vi "Write experiments.vi"(2 "error in (no error)":errorcluster, 3 "Experiments":refnum<class "Experiment.lvclass">[](array[class]), 4 "Experiments_group.lvclass in":refnum<class "Experiments_group.lvclass">) -> (0 "error out":errorcluster, 1 "Experiments_group.lvclass out":refnum<class "Experiments_group.lvclass">)   [LabVIEW 2019, in "Experiments_group.lvclass"]
uses:
  Experiments_group.lvclass
  Experiment.lvclass
  Experiments_group.lvclass/Experiments_group.ctl
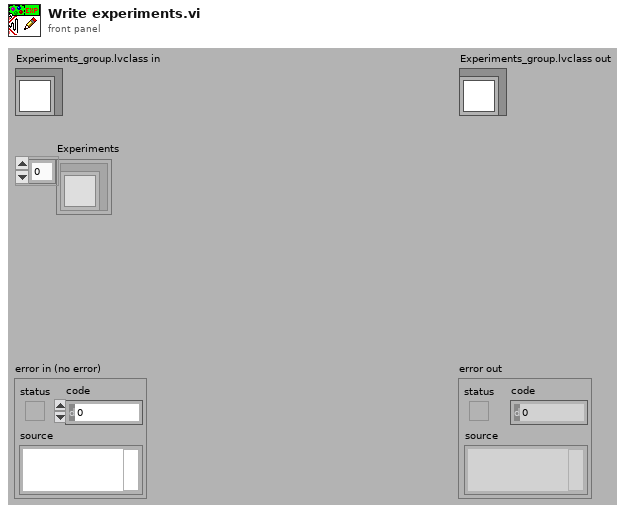
[diagram p1: front panel]
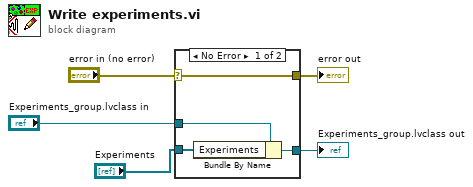
[diagram p0: block diagram]
diagram:
  n1 = case shown="No Error" "error in (no error)" {
    selector: "error in (no error)" -> [w9 w10]
    tunnel: [w9 w10] -> w4
    tunnel: [w8 w11] -> w2
    tunnel: "Experiments_group.lvclass in" -> [w6 w11]
    tunnel: "Experiments" -> [w7 _]
    frame No Error {
      n2 = Bundle By Name(cluster=w6, "Experiments"=w7) -> (w8:refnum<class "Experiments_group.lvclass">)
    }
    frame Error {
    }
  }
  "error out" <- w4
  "Experiments_group.lvclass out" <- w2
